vi "Next Step.vi"(8 "error in (no error)":errorcluster, 11 "Varian Continuous in":refnum<class "Varian Continuous.lvclass">) -> (0 "error out":errorcluster, 1 "Current Step":u32, 2 "Current Position":dbl, 3 "Varian Continuous out":refnum<class "Varian Continuous.lvclass">)   [LabVIEW 2009, in "Varian Continuous.lvclass"]
doc: "(Dynamic) Move to the next preconfigured step of this Scanner, and return the current position (actual, not intended) of this Scanner. Increment the step counter by one."
uses:
  Varian Continuous.lvclass
  Instruments/Varian Magnet/Varian Magnet.lvclass
  Scanner/Scanner.lvclass
  Instruments/Varian Magnet/Varian Max Field.vi
  Varian Continuous.lvclass/Varian Continuous.ctl
  <vilib>/DAQmx/create/channels.llb/DAQmx Create Channel (AO-Voltage-Basic).vi
  Global/GPIB Numbers.vi
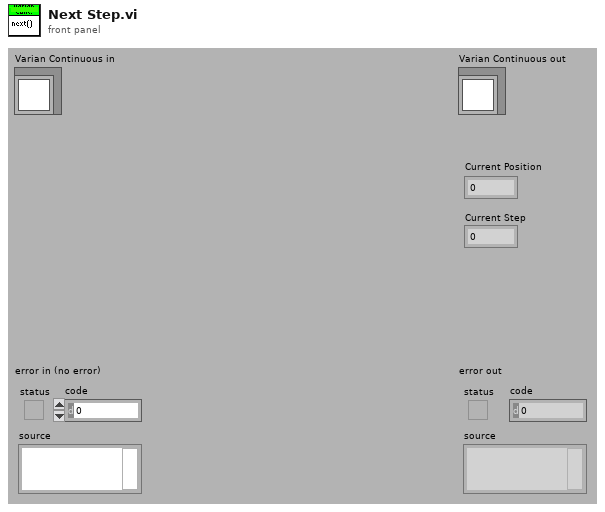
[diagram p1: front panel]
types:
  T1 = typedef "Scanner.lvclass/Range.ctl" = cluster{"xi":dbl, "xf":dbl, "dx":dbl, "Return to...?":bool, "Return to":dbl}
  T2 = typedef "GPIB Type Def.ctl" = cluster{"Name":string, "bus":dbl, "GPIB":dbl, "GPIB as string":string, "byte":i32, "VISA Resource Name":refnum<visa-resource-name>}
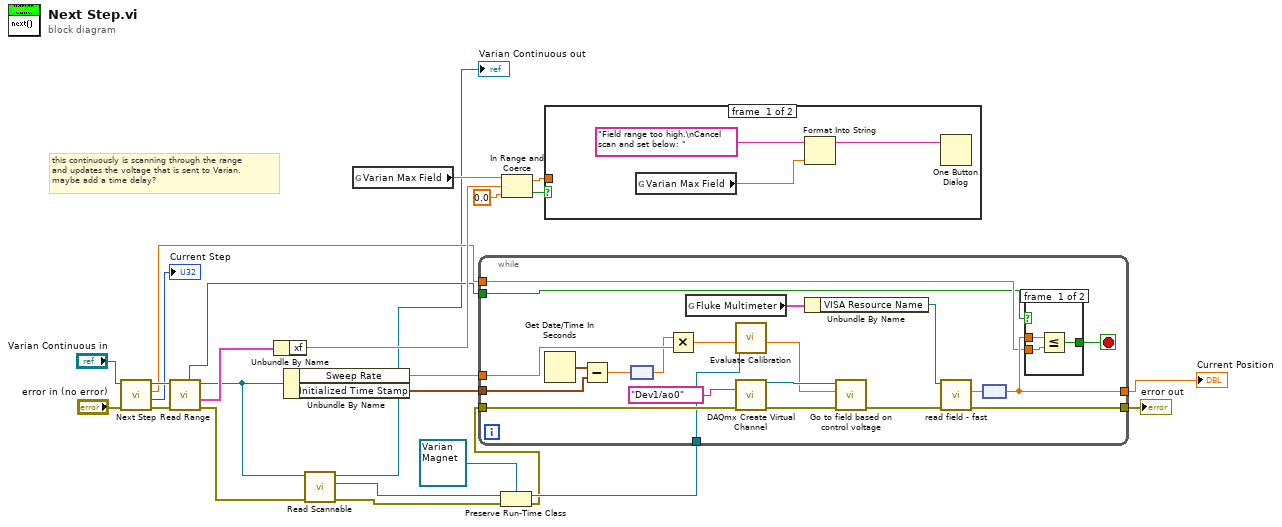
[diagram p0: block diagram]
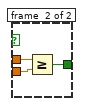
[diagram p2: hidden frame]
diagram:
  # "this continuously is scanning through the range\nand updates the voltage that is sent to Varian.\nmaybe add a time delay?"
  n1 = call-parent "Next Step.vi"("error in (no error)"="error in (no error)", "Scanner in"="Varian Continuous in") -> ("error out"=w20:errorcluster, "Current Step"=→"Current Step":u32, "Current Position"=w11:dbl, "Scanner out"=w21:refnum<class "Varian Continuous.lvclass">)  [unwired: 6 out]
  n2 = call-dynamic "Read Range.vi"("error in (no error)"=w20, "Scanner.lvclass in"=w21) -> ("error out"=w2:errorcluster, "Range"=w19:T1, "Scanner.lvclass out"=w8:refnum<class "Varian Continuous.lvclass">, "Scanning Up?"=w9:bool)  [unwired: 4 in, 2 out]
  n3 = Unbundle By Name(w19) -> ("xf"=w18:dbl)
  n4 = Unbundle By Name(w8) -> ("Sweep Rate"=w14:dbl[unit], "Initialized Time Stamp"=w15:timestamp)
  n5 = call-dynamic "Read Scannable.vi"("error in (no error)"=w2, "Scanner.lvclass in"=w8) -> ("error out"=w3:errorcluster, "Scannable.lvclass"=w5:refnum<class "Scannable.lvclass">, "Scanner.lvclass out"=→"Varian Continuous out":refnum<class "Varian Continuous.lvclass">)  [unwired: 7 in]
  n6 = global read "Varian Max Field.vi" "Varian Max Field"() -> (w23:dbl[unit])
  n7 = Preserve Run-Time Class(object in=w5, error in=w3, 2:refnum<class "Varian Magnet.lvclass"> refnum ("Varian Magnet.lvclass")) -> (object out=w4:refnum<class "Varian Magnet.lvclass">, error out=w1:errorcluster)
  n8 = while {
    tunnel: w15 -> [w41]
    tunnel: w14 -> [w31]
    tunnel: [w37] -> w12
    tunnel: w1 -> [w40]
    tunnel: [w39] -> w13
    tunnel: w11 -> [w36]
    tunnel: w9 -> [w34]
    tunnel: w4 -> [w26]
    stop <- w35 stop-if-true
    n9 = Get Date/Time In Seconds() -> (seconds since 1Jan1904=w42:timestamp)
    n10 = Subtract(x=w42, y=w41) -> (x-y=w30:dbl)
    n11 = node(w30) -> (w29:dbl[unit])
    n12 = Multiply(x=w29, y=w31) -> (x*y=w28:dbl[unit])
    n13 = global read "GPIB Numbers.vi" "Fluke Multimeter"() -> (w33:T2)
    n14 = call "Evaluate Calibration.vi"("tesla"=w28, "varian in"=w26) -> ("control voltage"=w27:dbl)  [unwired: 8 in, 1 out]
    n15 = call-poly <vilib>:"DAQmx Create Virtual Channel.vi"("physical channels"=tag "Dev1/ao0", "error in"=w40) -> ("task out"=w46:refnum<k21>, "error out"=w44:errorcluster)  [unwired: 7 in, 5 out]
    n16 = Unbundle By Name(w33) -> ("VISA Resource Name"=w32:refnum<visa-resource-name>)
    n17 = call "Go to field based on control voltage.vi"("error in"=w44, "Control Voltage"=w27, "task in"=w46) -> ("error out"=w45:errorcluster)  [unwired: 7 in, 1 out]
    n18 = call "read field - fast.vi"("error in (no error)"=w45, "VISA resource name"=w32) -> ("error out"=w39:errorcluster, "Current field (T)"=w38:dbl[unit])  [unwired: 7 in, 1 out]
    n19 = node(w38) -> (w37:dbl)
    n20 = case shown="True" w34 {
      tunnel: w37 -> [w48 w52]
      tunnel: w36 -> [w47 w51]
      tunnel: [w49 w50] -> w35
      frame #0 {
        n21 = Less Or Equal?(x=w48, y=w47) -> (x <= y?=w49:bool)
      }
      frame #1 {
        n22 = Greater Or Equal?(x=w52, y=w51) -> (x >= y?=w50:bool)
      }
    }
  }
  "error out" <- w13
  "Current Position" <- w12
  n23 = In Range and Coerce(upper limit=w23, x=w18, lower limit=dbl[unit] 0.0) -> (coerced(x)=w10:dbl[unit], In Range?=w17:bool)
  n24 = case shown="False" w17 {
    tunnel: w10 -> [_ _]
    frame #0 {
      n25 = global read "Varian Max Field.vi" "Varian Max Field"() -> (w53:dbl[unit])
      n26 = Format Into String(initial string="Field range too high.\nCancel scan and set below: " ("message"), w53) -> (resulting string=w55:string)  [unwired: 2 in, 1 out]
      n27 = One Button Dialog(message=w55) -> ()  [unwired: 1 in, 1 out]
    }
    frame #1 {
    }
  }
